vi "Connect Directional Ports.vi"(8 "error in":errorcluster, 10 "Digital Ports":tag[](array[tag]), 11 "6512 in":refnum<class "6512.lvclass">) -> (0 "error out":errorcluster, 3 "6512 out":refnum<class "6512.lvclass">)   [LabVIEW 2019, in "6512.lvlib" / "6512.lvclass"]
uses:
  Library/6512.lvclass
  C:/Users/Public/Documents/Development/builds/Instruments/DIG_IO.lvlibp/Library/DIG_IO.lvclass
  Library/6512.lvclass/6512.ctl
  Accessors/Read Local Resource.vi
  Accessors/Write Local Resource.vi
  builds/Instruments/DIG_IO.lvlibp/Accessors/Read BankDefs.vi
  <vilib>/DAQmx/create/channels.llb/DAQmx Create Channel (DO-Digital Output).vi
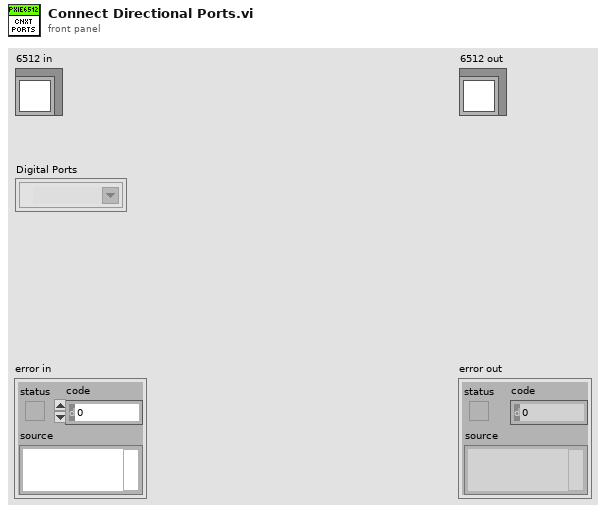
[diagram p1: front panel]
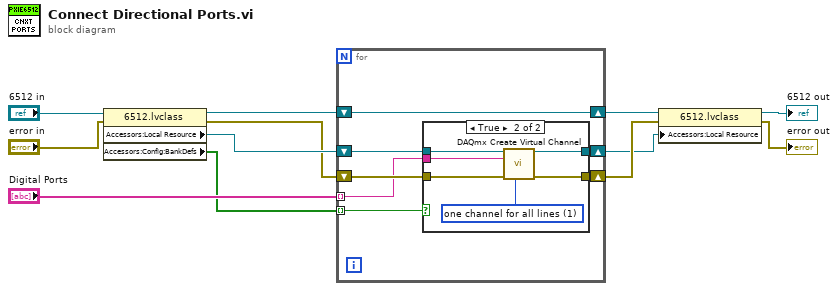
[diagram p0: block diagram]
diagram:
  n1 = property class="6512.lvclass"(reference="6512 in", error in="error in") -> (reference out=w10:refnum<class "6512.lvclass">, error out=w8:errorcluster, "Accessors:Local Resource"=w11:refnum<k21>, "Accessors:Config:BankDefs"=w1:bool[])
  n2 = for {
    shift-right: [w18] -> w3
    shift-left: w11 -> [w19]
    tunnel: "Digital Ports" -> [w14] mode=indexing
    shift-right: [w17] -> w5
    shift-left: w8 -> [w16]
    shift-right: [w15] -> w7
    shift-left: w10 -> [w15]
    tunnel: w1 -> [w13] mode=indexing
    n3 = case shown="True" w13 {
      tunnel: w19 -> [w21 w27]
      tunnel: [w21 w26] -> w18
      tunnel: [w20 w25] -> w17
      tunnel: w16 -> [w20 w24]
      tunnel: w14 -> [_ w22]
      frame False {
      }
      frame True {
        w23 = 1 items=["one channel for each line", "one channel for all lines"] ("line grouping")
        n4 = call-poly <vilib>:"DAQmx Create Virtual Channel.vi"("task in"=w27, "lines"=w22, "line grouping"=w23, "error in"=w24) -> ("task out"=w26:refnum<k21>, "error out"=w25:errorcluster)  [unwired: 10 in]
      }
    }
  }
  n5 = property class="6512.lvclass"(reference=w7, error in=w5, "Accessors:Local Resource"=w3) -> (reference out=→"6512 out":refnum<class "6512.lvclass">, error out=→"error out":errorcluster)
